vi "Sound.vi"(1 "error in (no error)":errorcluster, 2 "Base Path":path) -> (0 "error out":errorcluster)   [LabVIEW 2018]
doc: "Play the music.\nIt is dynamically called by Main.vi."
uses:
  <vilib>/sound2/lvsound2.llb/Sampling Mode.ctl
  Globals/Score.vi
  Globals/Stop.vi
  <vilib>/sound2/lvsound2.llb/Sound File Info (path).vi
  <vilib>/sound2/lvsound2.llb/Sound File Read Open.vi
  <vilib>/sound2/lvsound2.llb/Sound File Read (DBL).vi
  <vilib>/sound2/lvsound2.llb/Sound Output Write (DBL).vi
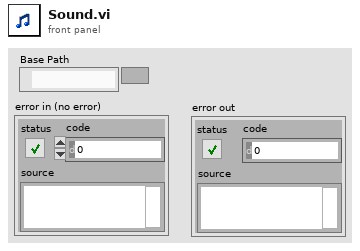
[diagram p1: front panel]
types:
  T1 = typedef "Sampling Mode.ctl" = i32
  T2 = typedef "Sound Data Format.ctl" = cluster{"sample rate (S/s)":dbl, "number of channels":i32, "bits per sample":i32}
  T3 = typedef "Sound File Refnum.ctl" = refnum<file>
  T4 = typedef "Sound Output Task ID.ctl" = u32
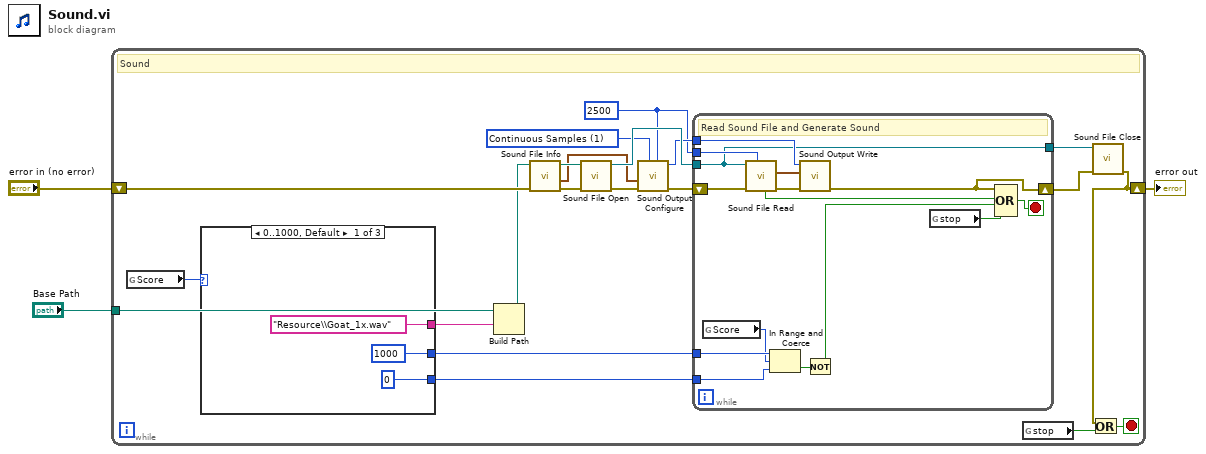
[diagram p0: block diagram]
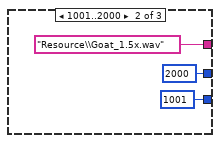
[diagram p2: hidden frame]
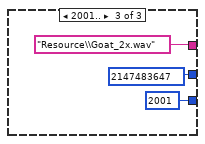
[diagram p3: hidden frame]
diagram:
  n1 = while {
    shift-right: [w6] -> w1
    shift-left: "error in (no error)" -> [w14]
    tunnel: "Base Path" -> [w5]
    stop <- w16 stop-if-true
    w17 = 2500
    w19 = T1 1 items=["Finite Samples", "Continuous Samples"] ("sample mode")
    # "Sound"
    n2 = global read "Score.vi" "Score"() -> (w7:i32)
    n3 = case shown="0..1000, Default" w7 {
      tunnel: ["Resource\\Goat_1x.wav" ("name or relative path") "Resource\\Goat_1.5x.wav" ("name or relative path") "Resource\\Goat_2x.wav" ("name or relative path")] -> w12
      tunnel: [1000 ("y") 2000 ("y") 2147483647 ("y")] -> w10
      tunnel: [0 1001 2001] -> w9
      frame 0..1000, Default {
      }
      frame 1001..2000 {
      }
      frame 2001.. {
      }
    }
    n4 = Build Path(base path=w5, name or relative path=w12) -> (appended path=w11:path)
    n5 = call-poly <vilib>:"Sound File Info.vi"("error in (no error)"=w14, "path"=w11) -> ("error out"=w23:errorcluster, "sound format"=w20:T2, "path out"=w21:path)  [unwired: 6 in, 1 out]
    n6 = call-poly <vilib>:"Sound File Open.vi"("error in (no error)"=w23, "path"=w21) -> ("error out"=w22:errorcluster, "sound file refnum"=w24:T3)  [unwired: 8 in]
    n7 = call <vilib>:"Sound Output Configure.vi"("number of samples/ch"=w17, "sample mode"=w19, "error in (no error)"=w22, "sound format"=w20) -> ("error out"=w15:errorcluster, "task ID"=w18:T4)  [unwired: 6 in]
    n8 = while {
      tunnel: w24 -> [w42]
      tunnel: w18 -> [w44]
      tunnel: w17 -> [w43]
      tunnel: [w42] -> w13
      shift-right: [w41] -> w8
      shift-left: w15 -> [w40]
      tunnel: w10 -> [w39]
      tunnel: w9 -> [w38]
      stop <- w46 stop-if-true
      # "Read Sound File and Generate Sound"
      n9 = global read "Score.vi" "Score"() -> (w35:i32)
      n10 = call-poly <vilib>:"Sound File Read.vi"("number of samples/ch (-1: all)"=w43, "error in (no error)"=w40, "sound file refnum"=w42) -> ("error out"=w48:errorcluster, "data"=w45:waveform(dbl)[], "end of file?"=w47:bool)  [unwired: 4 in, 2 out]
      n11 = In Range and Coerce(upper limit=w39, x=w35, lower limit=w38) -> (In Range?=w37:bool)  [unwired: 1 out]
      n12 = call-poly <vilib>:"Sound Output Write.vi"("error in (no error)"=w48, "data"=w45, "task ID"=w44) -> ("error out"=w41:errorcluster)  [unwired: 7 in, 1 out]
      n13 = Not(x=w37) -> (.not. x?=w36:bool)
      n14 = global read "Stop.vi" "stop"() -> (w34:bool)
      n15 = Compound Arithmetic op=OR(w41, w47, w36, w34) -> (w46:bool)
    }
    n16 = global read "Stop.vi" "stop"() -> (w4:bool)
    n17 = call <vilib>:"Sound File Close.vi"("error in (no error)"=w8, "sound file refnum"=w13) -> ("error out"=w6:errorcluster)  [unwired: 9 in]
    n18 = Or(x=w6, y=w4) -> (x .or. y?=w16:bool)
  }
  "error out" <- w1
